vi "AssignAndCount10.vi"(6 "Last region":bool=TRUE, 8 "Last laser bit in":bool, 9 "PMT bits in":bool[](array[boolean])=[FALSE, FALSE, FALSE, FALSE, FALSE, FALSE, FALSE, FALSE, FALSE, FALSE], 10 "Laser bits in":bool[](array[boolean])=[FALSE, FALSE, FALSE, FALSE, FALSE, FALSE, FALSE, FALSE, FALSE, FALSE], 11 "Photon counters in":T1=[0, 0]) -> (0 "New last laser bit out":bool, 3 "Photon counters out":T1, 4 "New last region out":bool)   [LabVIEW 2012]
uses:
  RegionalPhotonCounters.ctl
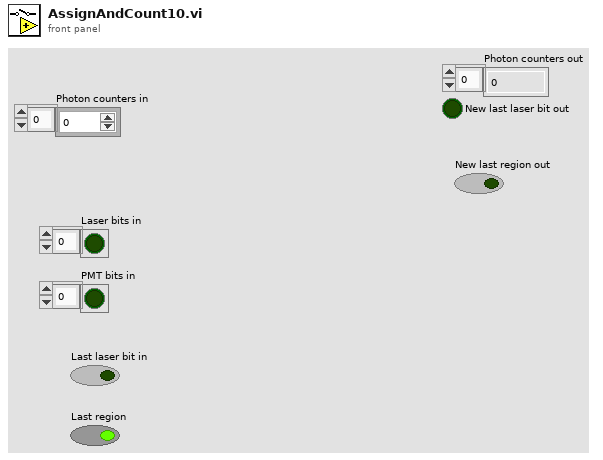
[diagram p1: front panel]
types:
  T1 = typedef "RegionalPhotonCounters.ctl" = i16[]
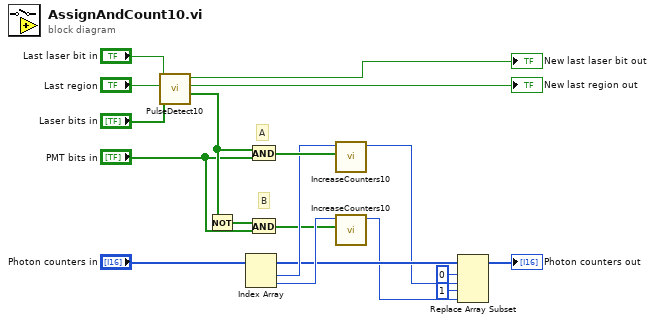
[diagram p0: block diagram]
diagram:
  # "B"
  # "A"
  n1 = call "PulseDetect10.vi"("Laser bits in"="Laser bits in", "Last region"="Last region", "Last laser bit in"="Last laser bit in") -> ("Region array out"=w15:bool[], "New last region out"=→"New last region out":bool, "New last laser bit out"=→"New last laser bit out":bool)  [unwired: 6 in]
  n2 = Not(x=w15) -> (.not. x?=w14:bool[])
  n3 = Index Array(array="Photon counters in") -> (element #1=w11:i16, element #2=w10:i16)  [unwired: 2 in]
  n4 = And(x=w15, y="PMT bits in") -> (x .and. y?=w12:bool[])
  n5 = And(x=w14, y="PMT bits in") -> (x .and. y?=w9:bool[])
  n6 = call "IncreaseCounters10.vi"("PMT pulses"=w12, "Counter in"=w11) -> ("Counter out"=w7:i16)  [unwired: 9 in]
  n7 = call "IncreaseCounters10.vi"("PMT pulses"=w9, "Counter in"=w10) -> ("Counter out"=w6:i16)  [unwired: 9 in]
  n8 = Replace Array Subset(array="Photon counters in", new element #1=w7, index #1=0 ("index"), new element #2=w6, index #2=1 ("index")) -> (→"Photon counters out":T1)
